vi "Get-lasing-data.vi"(8 "error in (no error)":errorcluster, 11 "Object ref in":T1) -> (0 "error out":errorcluster, 1 "Data":string, 2 "File name":string, 3 "Object ref out":T1)   [LabVIEW 2013, in "SLMControl.lvlib" / "SC-Main.lvclass"]
uses:
  SC-Main.lvclass
  Object-reference.ctl
  SC-Main.lvclass/SC-Main.ctl
  Read Lasing file index.vi
  Read Lasing files.vi
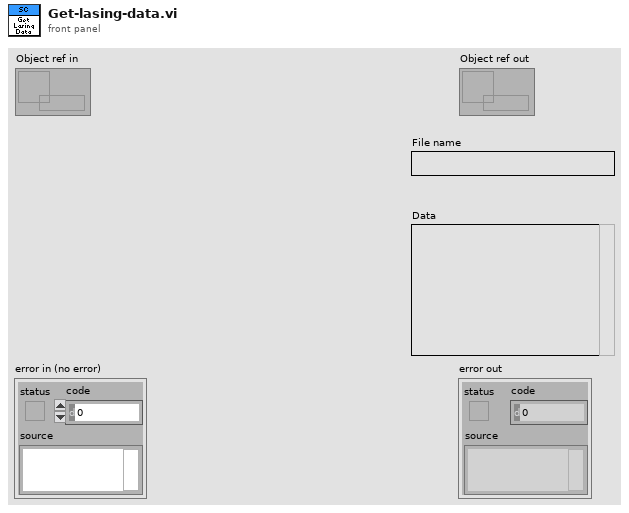
[diagram p1: front panel]
types:
  T1 = typedef "SLMControl.lvlib/SC-Main.lvclass/Object-reference.ctl" = refnum<data-value>
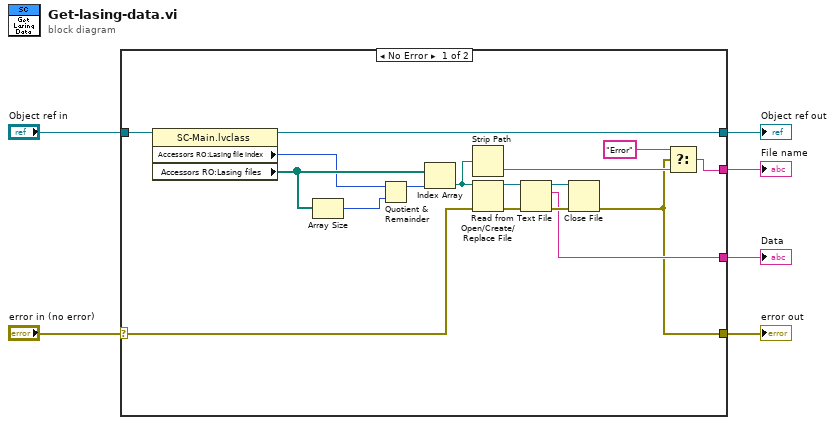
[diagram p0: block diagram]
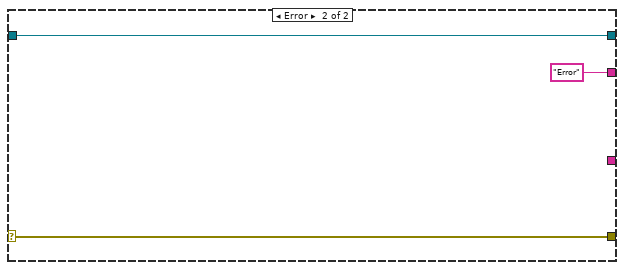
[diagram p2: hidden frame]
diagram:
  n1 = case shown="No Error" "error in (no error)" {
    selector: "error in (no error)" -> [w14 w26]
    tunnel: [w8 w26] -> w5
    tunnel: [w15 w25] -> w3
    tunnel: "Object ref in" -> [w16 w25]
    tunnel: [w13 _] -> w2
    tunnel: [w10 "Error" ("t")] -> w1
    frame No Error {
      n2 = property class="SC-Main.lvclass"(reference=w16) -> (reference out=w15:T1, "Accessors RO:Lasing file index"=w7:i32, "Accessors RO:Lasing files"=w21:path[])  [unwired: 1 in, 1 out]
      n3 = Array Size(array=w21) -> (size(s)=w22:i32)
      n4 = Quotient & Remainder(x=w7, y=w22) -> (x-y*floor(x/y)=w23:i32)  [unwired: 1 out]
      n5 = Index Array(array=w21, index=w23) -> (element=w12:path)
      n6 = Strip Path(path=w12) -> (name=w11:string)  [unwired: 1 out]
      n7 = Open/Create/Replace File(file path (use dialog)=w12, error in=w14) -> (refnum out=w17:refnum<file>, error out=w20:errorcluster)  [unwired: 4 in, 1 out]
      n8 = Read from Text File(file (use dialog)=w17, error in=w20) -> (refnum out=w18:refnum<file>, text=w13:string, error out=w19:errorcluster)  [unwired: 2 in, 1 out]
      n9 = Close File(refnum=w18, error in=w19) -> (error out=w8:errorcluster)  [unwired: 1 out]
      n10 = Select(t="Error", s=w8, f=w11) -> (s? t:f=w10:string)
    }
    frame Error {
    }
  }
  "error out" <- w5
  "Object ref out" <- w3
  "Data" <- w2
  "File name" <- w1
